vi "sendScript.vi"(8 "error in (no error)":errorcluster, 10 "runSingleScript":cluster{"Path":path, "HWLoop":bool}, 11 "ExperimentControl in":refnum<class "ExperimentControl.lvclass">) -> (0 "error out":errorcluster, 2 "configured":bool, 3 "ExperimentControl out":refnum<class "ExperimentControl.lvclass">)   [LabVIEW 2011, in "Views.lvlib" / "ExperimentControl.lvlib" / "ExperimentControl.lvclass"]
uses:
  ExperimentControl.lvclass
  ExperimentControl.lvclass/ExperimentControl.ctl
  Hal/HWController/HWControllerEvents/HWControllerEvents.lvclass
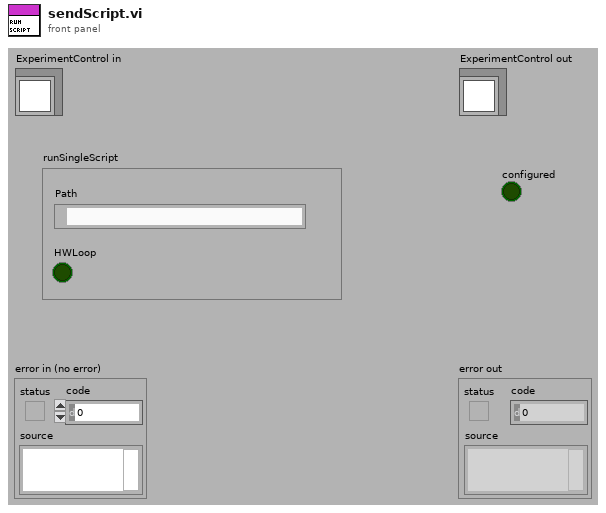
[diagram p1: front panel]
types:
  T1 = enum16{"start", "stop", "statusInquiry", "configure", "resetError", "resourcesInquiry", "reserveResources", "initialise", "resetAllChannels", "staticUpdate", "close", "HWStatus", "error", "resourcesAvailable", "resourcesReserved", "compilerError", "compiledScript", "compilingScript", "runScript", "configureCompiledScript"}
  T2 = enum16{"Ready", "Compiling", "Configured", "Running", "Stopping", "Unresolved Error"}
  T3 = cluster{"incomingEventTypes":cluster{"start":cluster{"Boolean":bool}, "stop":cluster{"Boolean":bool}, "statusInquiry":cluster{"Boolean":bool}, "configure":cluster{"DPScriptPath":path, "TimeStamp":string, "HWLoop?":bool}, "resetError":cluster{"Boolean":bool}, "resourcesInquiry":cluster{"Boolean":bool}, "reserveResources":cluster{"HWList":string[]}, "initialise":cluster{"HWList":string[]}, "close":cluster{"Boolean":bool}, "resetAllChannels":cluster{"Boolean":bool}, "staticChannelUpdate":cluster{"channel_address":string, "calibratedValue":dbl}, "runScript":cluster{"DPScriptPath":path, "TimeStamp":string, "HWLoop?":bool}, "compilingScript":cluster{"Path":path}, "compiledScript":cluster{"Path":path, "timeCompileAt":string}, "compilerError":cluster{"Path":path}, "configureCompiledScript":cluster{"DPScriptPath":path, "TimeStamp":string, "HWLoop?":bool, "CompiledScript":cluster{"ScriptListCompiler.lvclass":refnum<class "ScriptListCompiler.lvclass">, "aoChannels":refnum<class "AnalogOutput.lvclass">[], "doChannels":refnum<class "DigitalOutput.lvclass">[], "rfChannels":refnum<class "DDSOutput.lvclass">[]}}, "restartCompiler":cluster{"restart":bool}, "staticRfChannelUpdate":cluster{"channel_address":string, "Output":cluster{"Frequency(MHz)":dbl, "Amplitude":dbl, "Phase":dbl, "OutputForm":enum16{"Sine", "Square", "Triangle", "Arbitrary"}}}, "cameraUpdate":cluster{"Camera":string, "Type":string, "settings":path}}, "outgoingEventTypes":cluster{"HWStatus":cluster{"status":enum16{"Ready", "Compiling", "Configured", "Running", "Stopping", "Unresolved Error"}}, "error":cluster{"error out":errorcluster}, "resourcesAvailable":cluster{"availableHWList":string[], "reservedHWList":string[]}, "resourcesReserved":cluster{"reservedHWList":string[]}}}
  T4 = cluster{"DPScriptPath":path, "TimeStamp":string, "HWLoop?":bool}
  T5 = cluster{"eventId":enum16{"start", "stop", "statusInquiry", "configure", "resetError", "resourcesInquiry", "reserveResources", "initialise", "resetAllChannels", "staticUpdate", "close", "HWStatus", "error", "resourcesAvailable", "resourcesReserved", "compilerError", "compiledScript", "compilingScript", "runScript", "configureCompiledScript"}, "runScript":cluster{"DPScriptPath":path, "TimeStamp":string, "HWLoop?":bool}}
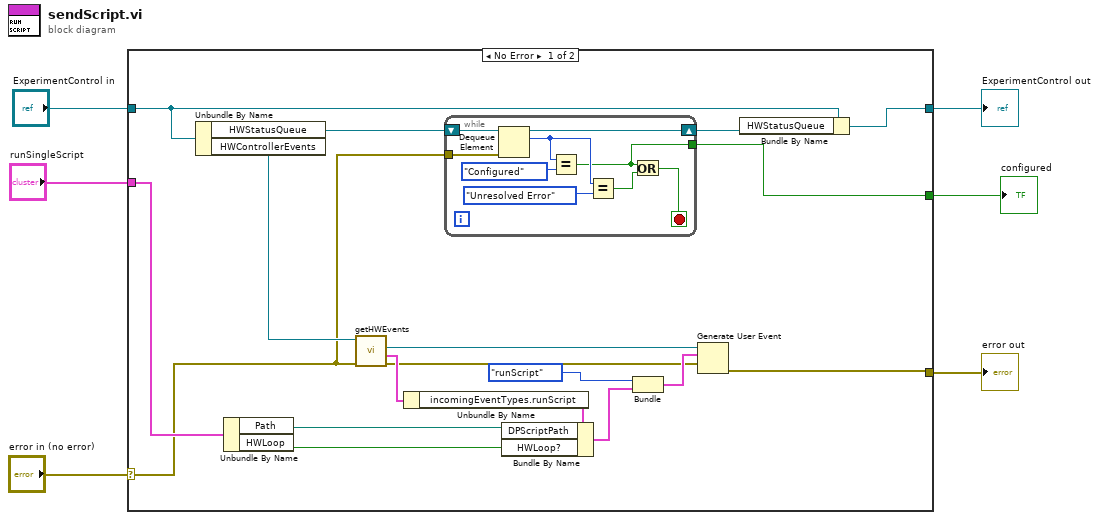
[diagram p0: block diagram]
diagram:
  n1 = case shown="No Error" "error in (no error)" {
    selector: "error in (no error)" -> [w13 w35]
    tunnel: [w10 w35] -> w5
    tunnel: [w8 w34] -> w3
    tunnel: "ExperimentControl in" -> [w9 w34]
    tunnel: "runSingleScript" -> [w17 _]
    tunnel: [w12 _] -> w1
    frame No Error {
      n2 = Unbundle By Name(w9) -> ("HWStatusQueue"=w14:refnum<queue>, "HWControllerEvents"=w24:refnum<class "HWControllerEvents.lvclass">)
      n3 = Unbundle By Name(w17) -> ("Path"=w16:path, "HWLoop"=w15:bool)
      n4 = call-dynamic "getHWEvents.vi"("error in (no error)"=w13, "HWControllerEvents in"=w24) -> ("error out"=w11:errorcluster, "eventDataTypes"=w18:T3, "HWCEvent"=w19:refnum<user-event>)  [unwired: 6 in, 1 out]
      n5 = Unbundle By Name(w18) -> ("incomingEventTypes.runScript"=w23:T4)
      n6 = while {
        tunnel: w13 -> [w32]
        shift-right: [w27] -> w7
        shift-left: w14 -> [w33]
        tunnel: [w25] -> w12
        stop <- w28 stop-if-true
        n7 = Dequeue Element(queue=w33, error in (no error)=w32) -> (queue out=w27:refnum<queue>, element=w30:T2)  [unwired: 1 in, 2 out]
        n8 = Equal?(x=w30, y=T2."Configured" ("element")) -> (x = y?=w25:bool)
        n9 = Equal?(x=w30, y=T2."Unresolved Error" ("element")) -> (x = y?=w26:bool)
        n10 = Or(x=w25, y=w26) -> (x .or. y?=w28:bool)
      }
      n11 = Bundle By Name(cluster=w23, "DPScriptPath"=w16, "HWLoop?"=w15) -> (w22:T4)
      n12 = Bundle("eventId"=T1."runScript", "runScript"=w22) -> (w20:T5)  [unwired: 1 in]
      n13 = Generate User Event(user event=w19, event data cluster=w20, error in=w11) -> (error out=w10:errorcluster)  [unwired: 1 out]
      n14 = Bundle By Name(cluster=w9, "HWStatusQueue"=w7) -> (w8:refnum<class "ExperimentControl.lvclass">)
    }
    frame Error {
    }
  }
  "error out" <- w5
  "ExperimentControl out" <- w3
  "configured" <- w1
